vi "RSNRPZ Get Scope Measurements Pulse Reference Levels.vi"(8 "error in (no error)":errorcluster, 10 "Channel (1)":i32=1, 11 "VISA session":refnum<visa-resource-name> caption="VISA resource name") -> (0 "error out":errorcluster, 1 "Low Ref Level":dbl format="%^.3e", 3 "dup VISA session":refnum<visa-resource-name> caption="VISA resource name", 4 "High Ref Level":dbl format="%^.3e", 5 "Duration Ref Level":dbl format="%^.3e")   [LabVIEW 2010]
doc: "This VI returns the calculated reference level in Watt at the defined thresholds of the last recorded trace. The thresholds in percent are defined with the VI rsnrpz_scope_meas_setLevelThresholds(…) of the pulse amplitude.\n\nNote:\n1) This VI is only available for NRP-Z81.\n\nRemote-control command(s):\nSENS:TRAC:MEAS:POW:LREF?\nSENS:TRAC:MEAS:POW:HREF?\nSENS:TRAC:MEAS:POW:REF?"
uses:
  rsnrpz_32.dll
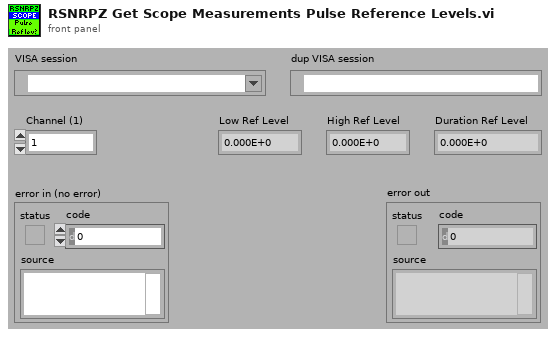
[diagram p1: front panel]
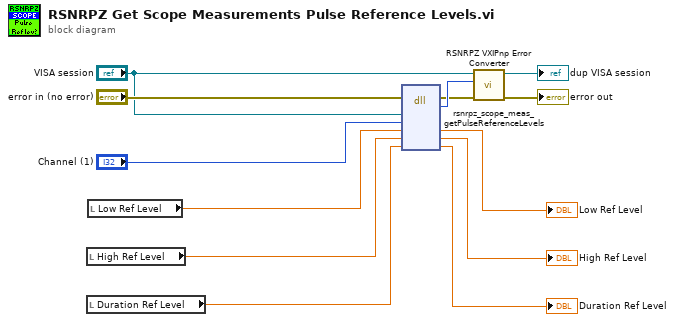
[diagram p0: block diagram]
diagram:
  n1 = local read "High Ref Level"() -> (w9:dbl)
  n2 = local read "Duration Ref Level"() -> (w7:dbl)
  n3 = local read "Low Ref Level"() -> (w11:dbl)
  n4 = dll-call lib="rsnrpz_32.dll" fn="rsnrpz_scope_meas_getPulseReferenceLevels"(error in="error in (no error)", "Instrument Handle"="VISA session", "Channel"="Channel (1)", "Low Ref Level"=w11, "High Ref Level"=w9, "Duration Ref Level"=w7) -> (error out=w5:errorcluster, "Status"=w13:i32, "Low Ref Level"=→"Low Ref Level":dbl, "High Ref Level"=→"High Ref Level":dbl, "Duration Ref Level"=→"Duration Ref Level":dbl)  [unwired: 4 in, 1 out]
  n5 = call <instrlib>:"RSNRPZ VXIPnp Error Converter.vi"("error in"=w5, "VXIPnp error code"=w13, "VISA session"="VISA session") -> ("error out"=→"error out":errorcluster, "dup VISA session"=→"dup VISA session":refnum<visa-resource-name>)  [unwired: 7 in]
